vi "CheckColision.vi"(8 "error in":errorcluster, 10 "AsterData":T2[](array[typedef]), 11 "ShootsData":T1[](array[typedef])) -> (0 "error out":errorcluster, 2 "AsterData out":T2[](array[typedef]), 3 "ShootsRefs out":T1[](array[typedef]))   [LabVIEW 2017]
uses:
  ManRef_ShootData.ctl
  ManRef_AsterData.ctl
  Spaceship/Shoot/Shoot_states.ctl
  Spaceship/Shoot/Shoot_data.ctl
  GameConfig/GameConfig_data.ctl
  Asteroid/Asteroid_states.ctl
  Asteroid/Asteroid_data.ctl
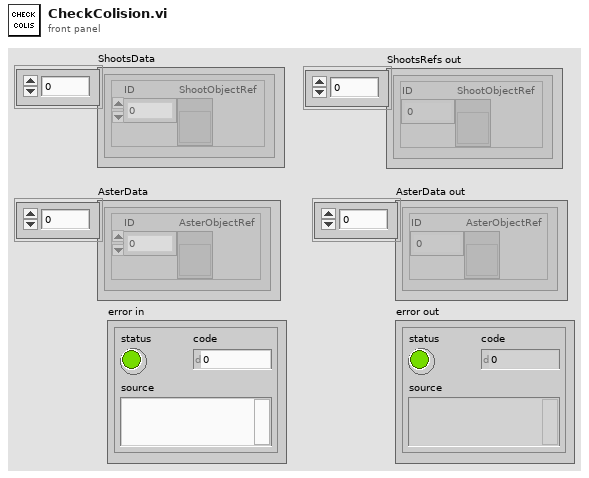
[diagram p1: front panel]
types:
  T1 = typedef "ManRef_ShootData.ctl" = cluster{"ID":i32, "ShootObjectRef":refnum<vi>}
  T2 = typedef "ManRef_AsterData.ctl" = cluster{"ID":i32, "AsterObjectRef":refnum<vi>}
  T3 = typedef "Shoot_data.ctl" = cluster{"Direction":dbl, "displayRef":refnum<vi>, "Max X":dbl, "Max Y":dbl, "Xpos":dbl, "Ypos":dbl, "ID":i32, "Config":T4}
  T4 = typedef "GameConfig_data.ctl" = cluster{"SpaceShip":cluster{"Angle":dbl, "SideLenght":dbl, "MaxLinearVeloc":dbl, "MaxAngularVeloc":dbl, "LinearAceleration":dbl, "AngularAceleration":dbl}, "Physics":cluster{"LinearDragFactor":dbl, "AngularDragFactor":dbl}, "Asteroids":cluster{"MaxSize":dbl, "MaxDivisions":i32, "MaxVeloc":dbl, "MinVeloc":dbl, "Fill":bool}, "Environment":cluster{"MaxAsteroids":i32, "TimeIncrement":dbl, "AsterProbCreation":dbl, "LogEnabled":bool}, "Shots":cluster{"MinTimeShots":dbl, "ShotSize":dbl, "ShotSpeed":dbl}}
  T5 = typedef "Shoot_states.ctl" = enum16{"Init", "Move", "Draw", "GetData", "Destroy"}
  T6 = typedef "Asteroid_data.ctl" = cluster{"Veloc":dbl, "Direction":dbl, "Size":i32, "displayRef":refnum<vi>, "Max X":dbl, "Max Y":dbl, "Xpos":dbl, "Ypos":dbl, "ID":i32, "Config":T4}
  T7 = typedef "Asteroid_states.ctl" = enum16{"Init", "Move", "Split", "GetData", "Draw", "Destroy"}
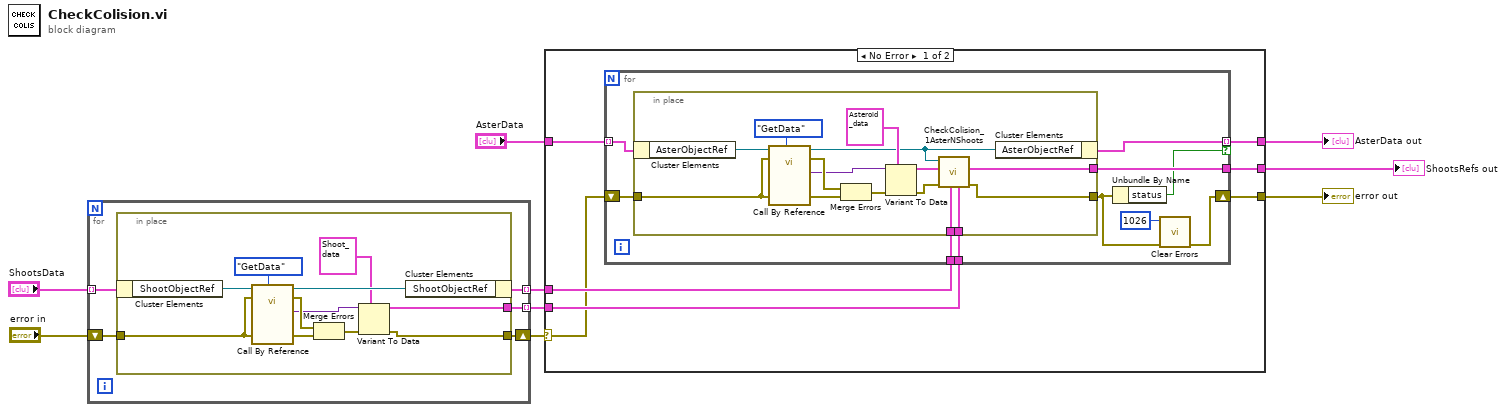
[diagram p0: block diagram]
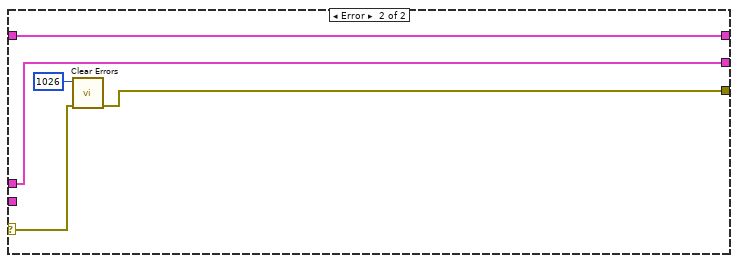
[diagram p2: hidden frame]
diagram:
  n1 = for {
    tunnel: "ShootsData" -> [w14] mode=indexing
    shift-right: [w12] -> w1
    shift-left: "error in" -> [w13]
    tunnel: [w11] -> w5 mode=indexing
    tunnel: [w10] -> w6 mode=indexing
    n2 = in-place {
      in-place-border: w13 -> [w24]
      in-place-border: [w16] -> w12
      in-place-border: [w15] -> w10
      n3 = in-place-cluster #1(w14) -> ("ShootObjectRef"=w25:refnum<vi>)
      n4 = call-by-ref "?"(reference=w25, error in=w24, "Shoot_states"=Shoot_states."GetData", "error in"=w24) -> (reference out=w23:refnum<vi>, error out=w20:errorcluster, 0:"error out"=w19:errorcluster, "DataOut"=w18:variant)  [unwired: 8 in]
      n5 = Merge Errors(w20, w19) -> (w21:errorcluster)
      n6 = Variant To Data(error in=w21, type=T3 {"Direction"=0.0, "displayRef"=refnum, "Max X"=0.0, "Max Y"=0.0, "Xpos"=0.0, "Ypos"=0.0, "ID"=0, "Config"={"SpaceShip"={"Angle"=30.0, "SideLenght"=2.0, "MaxLinearVeloc"=10.0, "MaxAngularVeloc"=10.0, "LinearAceleration"=1.0, "AngularAceleration"=1.0}, "Physics"={"LinearDragFactor"=1.0, "AngularDragFactor"=1.0}, "Asteroids"={"MaxSize"=6.0, "MaxDivisions"=3, "MaxVeloc"=8.0, "MinVeloc"=1.0, "Fill"=FALSE}, "Environment"={"MaxAsteroids"=10, "TimeIncrement"=0.1, "AsterProbCreation"=0.1, "LogEnabled"=FALSE}, "Shots"={"MinTimeShots"=10.0, "ShotSize"=0.1, "ShotSpeed"=0.1}}} ("ShootData"), Variant=w18) -> (data=w15:T3, error out=w16:errorcluster)
      n7 = in-place-cluster #1("ShootObjectRef"=w23) -> (w11:T1)
    }
  }
  n8 = case shown="No Error" w1 {
    selector: w1 -> [w26 w59]
    tunnel: "AsterData" -> [w32 w62]
    tunnel: w6 -> [w31 _]
    tunnel: w5 -> [w30 w61]
    tunnel: [w29 w58] -> w4
    tunnel: [w28 w62] -> w3
    tunnel: [w27 w61] -> w2
    frame No Error {
      n9 = for {
        tunnel: w32 -> [w42] mode=indexing
        shift-right: [w33] -> w29
        shift-left: w26 -> [w41]
        tunnel: [w40] -> w28 mode=indexing if=w36
        tunnel: w31 -> [w38]
        tunnel: w30 -> [w39]
        tunnel: [w37] -> w27
        n10 = in-place {
          in-place-border: w41 -> [w56]
          in-place-border: [w46] -> w34
          in-place-border: w39 -> [w45]
          in-place-border: w38 -> [w44]
          in-place-border: [w43] -> w37
          n11 = in-place-cluster #2(w42) -> ("AsterObjectRef"=w57:refnum<vi>)
          n12 = call-by-ref "?"(reference=w57, error in=w56, "Asteroid_states"=Asteroid_states."GetData", "error in"=w56) -> (reference out=w48:refnum<vi>, error out=w53:errorcluster, 0:"error out"=w54:errorcluster, "DataOut"=w51:variant)  [unwired: 8 in]
          n13 = Merge Errors(w53, w54) -> (w52:errorcluster)
          n14 = Variant To Data(error in=w52, type=T6 {"Veloc"=0.0, "Direction"=0.0, "Size"=0, "displayRef"=refnum, "Max X"=0.0, "Max Y"=0.0, "Xpos"=0.0, "Ypos"=0.0, "ID"=0, "Config"={"SpaceShip"={"Angle"=30.0, "SideLenght"=2.0, "MaxLinearVeloc"=10.0, "MaxAngularVeloc"=10.0, "LinearAceleration"=1.0, "AngularAceleration"=1.0}, "Physics"={"LinearDragFactor"=1.0, "AngularDragFactor"=1.0}, "Asteroids"={"MaxSize"=6.0, "MaxDivisions"=3, "MaxVeloc"=8.0, "MinVeloc"=1.0, "Fill"=FALSE}, "Environment"={"MaxAsteroids"=10, "TimeIncrement"=0.1, "AsterProbCreation"=0.1, "LogEnabled"=FALSE}, "Shots"={"MinTimeShots"=10.0, "ShotSize"=0.1, "ShotSpeed"=0.1}}} ("AsteroidData"), Variant=w51) -> (data=w49:T6, error out=w47:errorcluster)
          n15 = call "CheckColision_1AsterNShoots.vi"("ShootsData"=w44, "ShootsRefs"=w45, "Error In"=w47, "AsterData"=w49, "RefAster"=w48) -> ("Error Out"=w46:errorcluster, "ShootsRefs out"=w43:T1[])  [unwired: 5 in]
          n16 = in-place-cluster #2("AsterObjectRef"=w48) -> (w40:T2)
        }
        n17 = Unbundle By Name(w34) -> ("status"=w36:bool)
        n18 = call <vilib>:"Clear Errors.vi"("error in (no error)"=w34, "specific error code to clear (0: all)"=1026) -> ("error out"=w33:errorcluster)  [unwired: 4 in, 1 out]
      }
    }
    frame Error {
      n19 = call <vilib>:"Clear Errors.vi"("error in (no error)"=w59, "specific error code to clear (0: all)"=1026) -> ("error out"=w58:errorcluster)  [unwired: 4 in, 1 out]
    }
  }
  "error out" <- w4
  "AsterData out" <- w3
  "ShootsRefs out" <- w2
